vi "convert_list2string.vi"(0 "LIST":string[](array[string]), 2 "BEGIN (CHAR)":string, 3 "CLUSTER (CHAR)":string, 4 "SEPARATOR (CHAR)":string, 5 "TERM (CHAR)":string) -> (14 "RESULT":string)   [LabVIEW 2018, in "db_lib R3.lvlib"]
uses:
  db_lib R3.lvlib
panel:
  # "Result string:\n[begin] [cluster] [data(0)] [cluster] [separator]\n[cluster] [data(1)] [cluster] [separator]\n[cluster] data(n)] [cluster] [termination]"
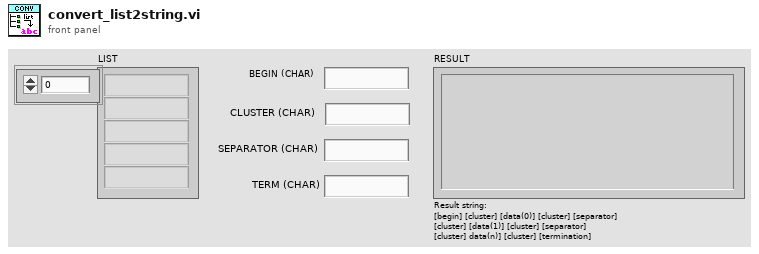
[diagram p1: front panel]
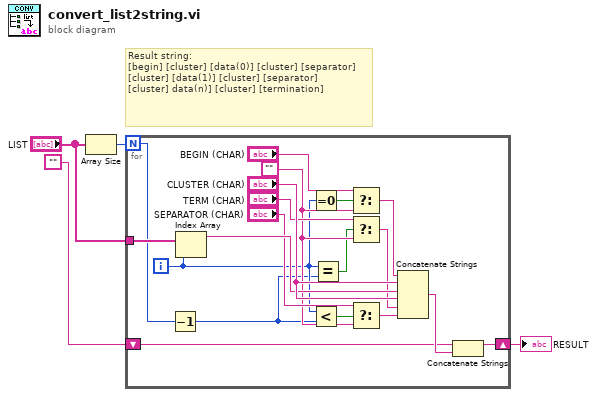
[diagram p0: block diagram]
diagram:
  # "Result string:\n[begin] [cluster] [data(0)] [cluster] [separator]\n[cluster] [data(1)] [cluster] [separator]\n[cluster] data(n)] [cluster] [termination]"
  n1 = Array Size(array="LIST") -> (size(s)=w4:i32)
  n2 = for {
    N: w4 -> [w19]
    tunnel: "LIST" -> [w20]
    shift-right: [w13] -> w1
    shift-left: "" -> [w12]
    i -> [w7]
    w9 = ""
    n3 = Decrement(x=w19) -> (x-1=w6:i32)
    n4 = Index Array(array=w20, index=w7) -> (element=w18:string)
    n5 = Equal To 0?(x=w7) -> (x = 0?=w22:bool)
    n6 = Less?(x=w7, y=w6) -> (x < y?=w8:bool)
    n7 = Equal?(x=w7, y=w6) -> (x = y?=w5:bool)
    n8 = Select(t="BEGIN (CHAR)", s=w22, f=w9) -> (s? t:f=w16:string)
    n9 = Select(t="TERM (CHAR)", s=w5, f=w9) -> (s? t:f=w15:string)
    n10 = Select(t="SEPARATOR (CHAR)", s=w8, f=w9) -> (s? t:f=w10:string)
    n11 = Concatenate Strings(w16, "CLUSTER (CHAR)", w18, "CLUSTER (CHAR)", w15, w10) -> (w14:string)
    n12 = Concatenate Strings(w12, w14) -> (w13:string)
  }
  "RESULT" <- w1
